vi "创建实例与初始化.vi"(7 "运算":T1, 8 "error in (no error)":errorcluster caption="错误输入（无错误）", 9 "B":dbl, 10 "A":dbl, 11 "运算工厂 输入":refnum<class "运算工厂.lvclass"> caption="DNL_LabVIEW Object in") -> (0 "error out":errorcluster caption="错误输出", 1 "结果":dbl, 2 "运算类 输出":refnum<class "运算类.lvclass">, 3 "运算工厂 输出":refnum<class "运算工厂.lvclass"> caption="DNL_LabVIEW Object out")   [LabVIEW 2013, in "运算工厂.lvclass"]
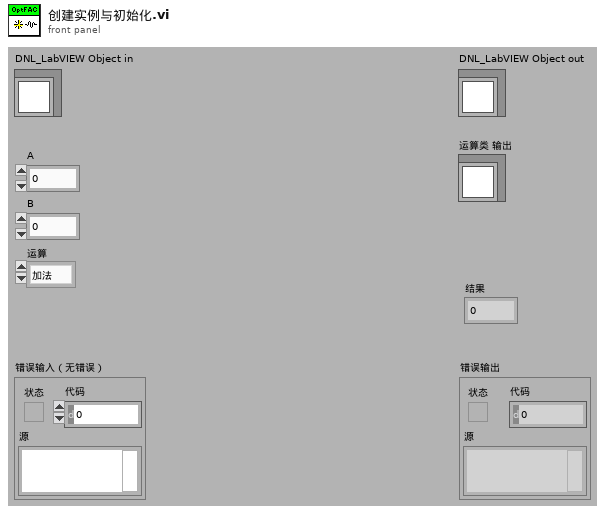
[diagram p1: front panel]
types:
  T1 = typedef "运算工厂.lvclass/运算方法.ctl" = enum16{"加法", "减法", "乘法", "平方和"}
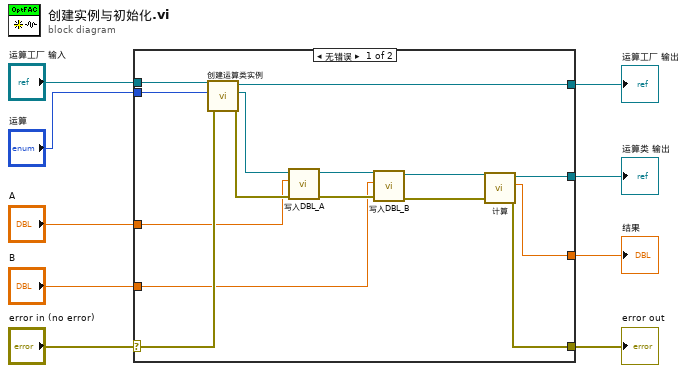
[diagram p0: block diagram]
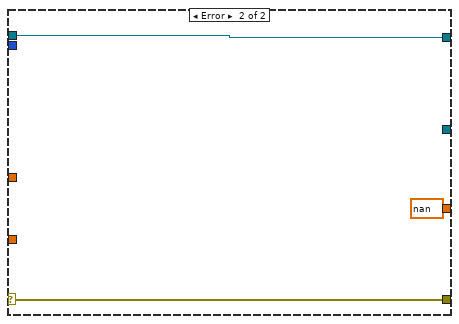
[diagram p2: hidden frame]
diagram:
  n1 = case shown="无错误" "error in (no error)" {
    selector: "error in (no error)" -> [w21 w27]
    tunnel: [w11 w27] -> w8
    tunnel: [w23 w26] -> w6
    tunnel: "运算工厂 输入" -> [w24 w26]
    tunnel: "运算" -> [w22 _]
    tunnel: "A" -> [w17 _]
    tunnel: "B" -> [w15 _]
    tunnel: [w12 nan ("结果")] -> w2
    tunnel: [w10 _] -> w1
    frame No Error {
      n2 = call "创建运算类实例.vi"("error in (no error)"=w21, "运算"=w22, "运算工厂 输入"=w24) -> ("error out"=w19:errorcluster, "运算类.lvclass"=w20:refnum<class "运算类.lvclass">, "运算工厂 输出"=w23:refnum<class "运算工厂.lvclass">)  [unwired: 6 in]
      n3 = call "写入DBL_A.vi"("error in (no error)"=w19, "DBL_A"=w17, "运算类输入"=w20) -> ("error out"=w18:errorcluster, "运算类输出"=w16:refnum<class "运算类.lvclass">)  [unwired: 7 in]
      n4 = call "写入DBL_B.vi"("error in (no error)"=w18, "DBL_B"=w15, "运算类输入"=w16) -> ("error out"=w14:errorcluster, "运算类输出"=w13:refnum<class "运算类.lvclass">)  [unwired: 7 in]
      n5 = call-dynamic "计算.vi"("error in (no error)"=w14, "运算类 输入"=w13) -> ("error out"=w11:errorcluster, "结果"=w12:dbl, "运算类 输出"=w10:refnum<class "运算类.lvclass">)  [unwired: 7 in]
    }
    frame Error {
    }
  }
  "error out" <- w8
  "运算工厂 输出" <- w6
  "结果" <- w2
  "运算类 输出" <- w1
